vi "golde_version_check.vi"() -> ()   [LabVIEW 2017]
panel:
  out "Out":u8=3 format="%.0x"
  out "error out":errorcluster
  in  "address":string="192.168.10.34"
  in  "error in (no error)":errorcluster
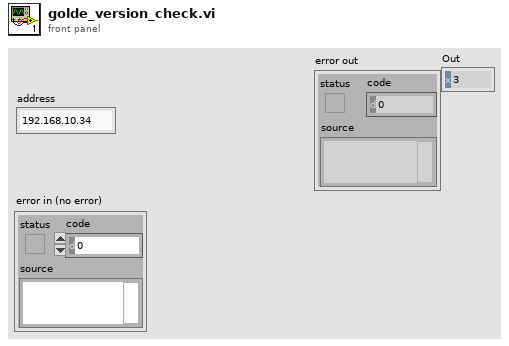
[diagram p1: front panel]
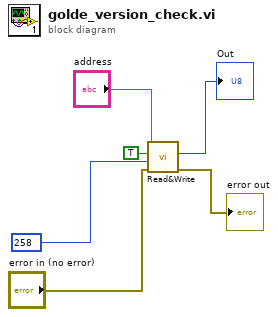
[diagram p0: block diagram]
diagram:
  n1 = call "Read&Write.vi"("error in (no error)"="error in (no error)", "Address"=u32 258, "Read (TRUE)"=TRUE, "address"="address") -> ("error out"=→"error out":errorcluster, "Out"=→"Out":u8)  [unwired: 6 in]
